vi "Define Target.vi"(8 "error in (no error)":errorcluster, 10 "Target Enqueuer":refnum<class "Message Enqueuer.lvclass">, 11 "Targetted Msg in":refnum<class "Bypass Msg.lvclass">) -> (0 "error out":errorcluster, 3 "Targetted Msg out":refnum<class "Bypass Msg.lvclass">)   [LabVIEW 2020, in "Publisher.lvlib" / "Bypass Msg.lvclass"]
doc: "Configure 'Bypass Msg' for execution."
uses:
  Bypass Msg.lvclass
  PPL/HDH.Actor Framework.Core.Actor.lvlibp/1abvi3w/vi.lib/ActorFramework/Message Enqueuer/Message Enqueuer.lvclass
  Bypass Msg.lvclass/Bypass Msg.ctl
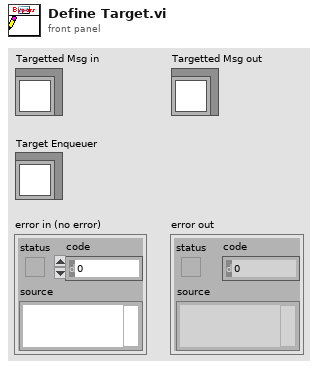
[diagram p1: front panel]
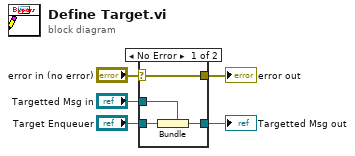
[diagram p0: block diagram]
diagram:
  n1 = case shown="No Error" "error in (no error)" {
    selector: "error in (no error)" -> [w7 w10]
    tunnel: [w7 w10] -> w4
    tunnel: [w9 w11] -> w2
    tunnel: "Targetted Msg in" -> [w6 w11]
    tunnel: "Target Enqueuer" -> [w8 _]
    frame No Error {
      n2 = Bundle(cluster=w6, w8) -> (w9:refnum<class "Bypass Msg.lvclass">)
    }
    frame Error {
    }
  }
  "error out" <- w4
  "Targetted Msg out" <- w2
